vi "Reset Error.vi"(8 "error in (no error)":errorcluster, 11 "FHPP in":refnum<class "FHPP.lvclass">) -> (0 "error out":errorcluster, 3 "FHPP out":refnum<class "FHPP.lvclass">)   [LabVIEW 2022 SP3, in "FHPP.lvclass"]
uses:
  FHPP.lvclass
  FHPP.lvclass/FHPP.ctl
  287bf636-282c-49fa-822a-e79821efdea6.vi
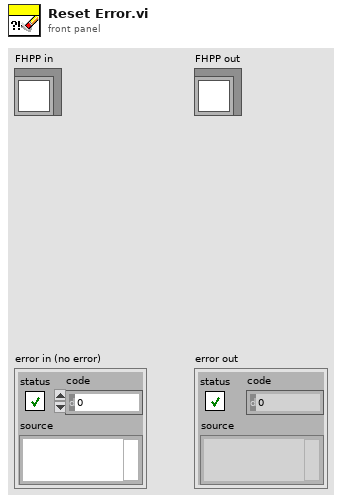
[diagram p1: front panel]
types:
  T1 = typedef "FHPP.lvclass/CCON.ctl" = cluster{"Enabled Drive":bool, "Stop":bool, "Open Brake":bool, "Reset Fault":bool, "Reserved":bool, "Lock Software Access":bool, "Operating Mode":T2}
  T2 = typedef "FHPP.lvclass/Operating Mode.ctl" = enum16{"Record Selection", "Direct Mode", "Reserved 1", "Reserved 2"}
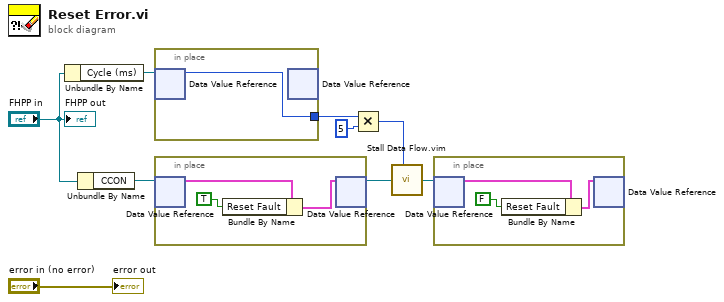
[diagram p0: block diagram]
diagram:
  n1 = Unbundle By Name("FHPP in") -> ("Cycle (ms)"=w4:refnum<data-value>)
  n2 = Unbundle By Name("FHPP in") -> ("CCON"=w8:refnum<data-value>)
  n3 = in-place {
    in-place-border: [w10] -> w3
    n4 = in-place-dvr #1(w4) -> (w10:i32)  [unwired: 1 out]
    n5 = in-place-dvr #1() -> ()  [unwired: 1 in, 2 out]
  }
  n6 = in-place {
    n7 = in-place-dvr #2(w8) -> (w13:T1)  [unwired: 1 out]
    n8 = Bundle By Name(cluster=w13, "Reset Fault"=TRUE) -> (w12:T1)
    n9 = in-place-dvr #2(w12) -> (w7:refnum<data-value>)  [unwired: 1 out]
  }
  n10 = Multiply(x=w3, y=5) -> (x*y=w1:i32)
  n11 = call "Stall Data Flow.vim"("value in"=w7, "milliseconds to wait"=w1) -> ("value out"=w6:refnum<data-value>)  [unwired: 1 out]
  n12 = in-place {
    n13 = in-place-dvr #3(w6) -> (w16:T1)  [unwired: 1 out]
    n14 = Bundle By Name(cluster=w16, "Reset Fault"=FALSE) -> (w15:T1)
    n15 = in-place-dvr #3(w15) -> ()  [unwired: 2 out]
  }
  "error out" <- "error in (no error)"
  "FHPP out" <- "FHPP in"
